vi "mapEventCounts.vi"(5 "Count":u32[](array[numeric])) -> (1 "Counts (map)":map{u32, u32}(c390), 2 "Count Grid":u32[][](array[numeric]))   [LabVIEW 2019]
uses:
  <vilib>/Utility/miscctls.llb/LVMapReplaceAction.ctl
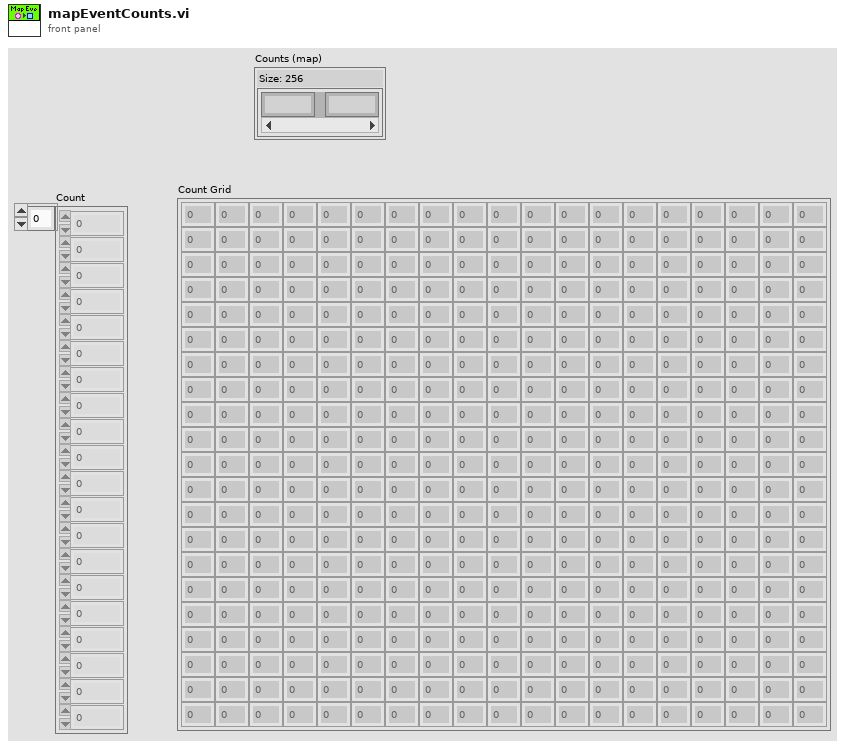
[diagram p1: front panel]
types:
  T1 = typedef "LVMapReplaceAction.ctl" = enum32{"Modify Entry only if found", "Add or Modify Entry", "Delete Entry"}
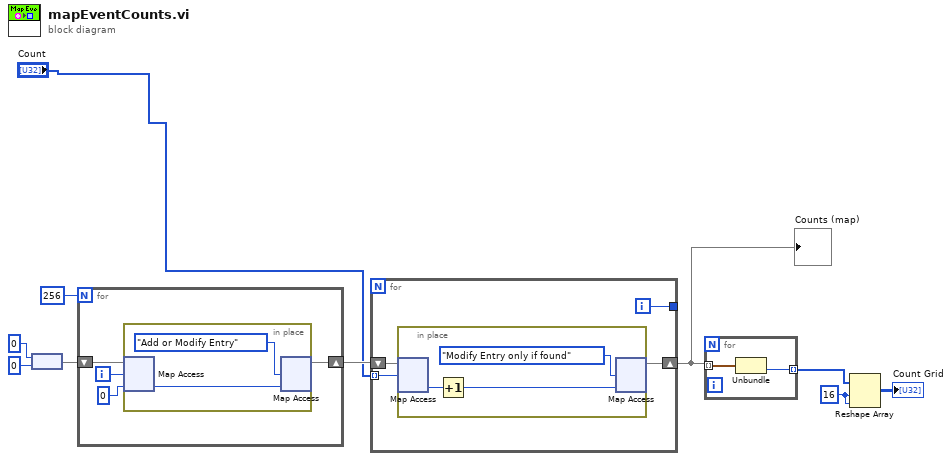
[diagram p0: block diagram]
diagram:
  w10 = 16
  n1 = node(u32 0, u32 0 ("value")) -> (w4:map{u32, u32})
  n2 = for {
    N: 256 -> [_]
    shift-right: [w11] -> w8
    shift-left: w4 -> [w14]
    i -> [w13]
    n3 = in-place {
      n4 = in-place-map #1(w14, w13, 0) -> (w15:u32)  [unwired: 1 out]
      n5 = in-place-map #1(w15, LVMapReplaceAction."Add or Modify Entry" ("action")) -> (w11:map{u32, u32})  [unwired: 2 out]
    }
  }
  n6 = for {
    shift-right: [w19] -> w1
    shift-left: w8 -> [w20]
    tunnel: "Count" -> [w18] mode=indexing
    tunnel: [w17] -> _
    i -> [w17]
    n7 = in-place {
      n8 = in-place-map #2(w20, w18) -> (w22:u32)  [unwired: 1 in, 1 out]
      n9 = Increment(x=w22) -> (x+1=w21:u32)
      n10 = in-place-map #2(w21, LVMapReplaceAction."Modify Entry only if found" ("action")) -> (w19:map{u32, u32})  [unwired: 2 out]
    }
  }
  "Counts (map)" <- w1
  n11 = for {
    tunnel: w1 -> [w25] mode=indexing
    tunnel: [w24] -> w9 mode=indexing
    n12 = Unbundle(w25) -> ("value"=w24:u32)  [unwired: 1 out]
  }
  n13 = Reshape Array(w9, w10, w10) -> (→"Count Grid":u32[][])
